vi "TestTimetoString.vi"() -> ()   [LabVIEW 2015]
panel:
  out "x = y?":bool
  out "Time Stamp 2":timestamp
  out "x-y":dbl
  out "Pass 2":bool
  out "Time Stamp":timestamp
  out "current time":timestamp
  out "error out":errorcluster
  out "Pass":bool
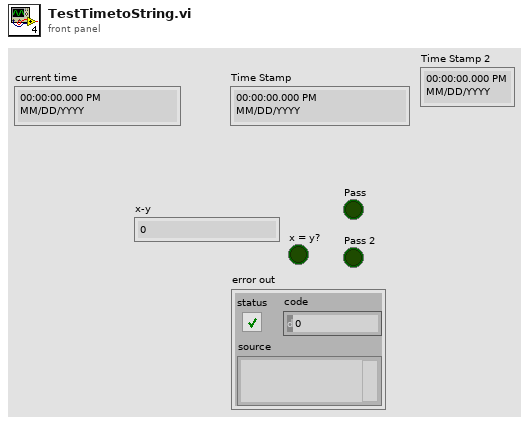
[diagram p1: front panel]
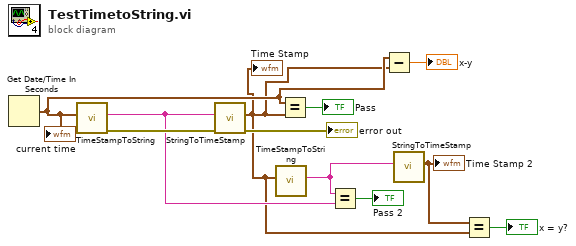
[diagram p0: block diagram]
diagram:
  n1 = Get Date/Time In Seconds() -> (seconds since 1Jan1904=w6:timestamp)
  "current time" <- w6
  n2 = call "TimeStampToString.vi"("Time Stamp"=w6) -> ("error out"=w10:errorcluster, "String"=w7:string)  [unwired: 9 in]
  n3 = call "StringToTimeStamp.vi"("error in (no error)"=w10, "TimeStamp"=w7) -> ("error out"=→"error out":errorcluster, "Time Stamp"=w2:timestamp)  [unwired: 8 in]
  "Time Stamp" <- w2
  n4 = call "TimeStampToString.vi"("Time Stamp"=w2) -> ("String"=w4:string)  [unwired: 9 in, 1 out]
  n5 = Equal?(x=w6, y=w2) -> (x = y?=→"Pass":bool)
  n6 = Equal?(x=w4, y=w7) -> (x = y?=→"Pass 2":bool)
  n7 = Subtract(x=w6, y=w2) -> (x-y=→"x-y":dbl)
  n8 = call "StringToTimeStamp.vi"("TimeStamp"=w4) -> ("Time Stamp"=w3:timestamp)  [unwired: 9 in, 1 out]
  "Time Stamp 2" <- w3
  n9 = Equal?(x=w3, y=w2) -> (x = y?=→"x = y?":bool)
